vi "UDP Multicast Sender.vi"() -> ()   [LabVIEW 2010]
doc: "Designed to work with the UDP Multicast Receiver.vi. Run the UDP Multicast Receiver.vi first.\n\nUDP multicast will allow LabVIEW to send data to a multicast group or to receive data sent to a multicast group. In LabVIEW, UDP multicast is used in very much the same way as UDP. The main difference is there are two new parameters, TTL and Multicast Address, on the UDP Multicast Open. \n\nWhen sending to a multicast group the default time-to-live (TTL) is 1, which only allows the packet to go to the local subnet. When a router receives a multicast packet, it decrements the packets TTL, and if the TTL is greater than 0, forwards the packet to other routers.\nA multicast group is defined by having a multicast IP address in the range 224.0.0.0 to 239.255.255.255."
uses:
  <vilib>/Utility/tcp.llb/UDP Multicast Open.vi
panel:
  in  "milliseconds to wait":u32=50
  in  "stop":bool
  in  "Multicast Address":string="234.5.6.7"
  in  "Data String":string="UDP Multicast Sender Data"
  in  "Send to Port":u16=58432
  in  "Local Port":u16=58431
  in  "TTL":u16=2
  # "Instructions:\n1. Open the UDP Multicast Receiver.vi located in the same library.\n2. Make sure that Remote Port in this VI and Port in the UDP Multicast Receiver.vi are the same and that they have the same Multicast Address.\n3. Follow the instructions on it's front panel.\nNote: This VI is built to work with the UDP Multicast Receiver.vi."
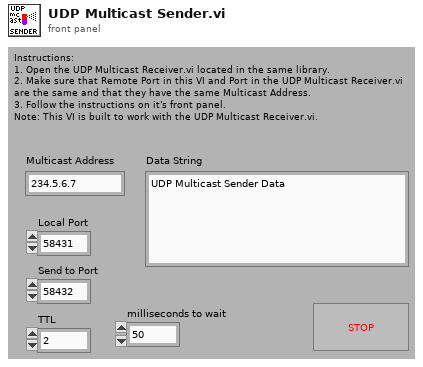
[diagram p1: front panel]
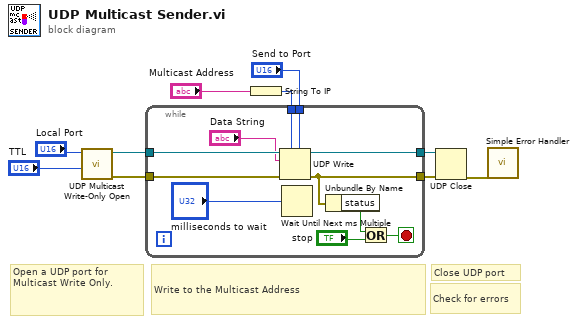
[diagram p0: block diagram]
diagram:
  # "Check for errors"
  # "Close UDP port"
  # "Write to the Multicast Address"
  # "Open a UDP port for Multicast Write Only."
  n1 = call-poly <vilib>:"UDP Multicast Write-Only Open.vi"("time-to-live (1)"="TTL", "port"="Local Port") -> ("error out"=w8:errorcluster, "connection ID"=w10:refnum<k16>)  [unwired: 8 in]
  n2 = String To IP(1:"Multicast Address") -> (0:w5:u32)
  n3 = while {
    tunnel: w10 -> [w21]
    tunnel: [w20] -> w9
    tunnel: w8 -> [w19]
    tunnel: [w12] -> w7
    tunnel: "Send to Port" -> [w18]
    tunnel: w5 -> [w17]
    stop <- w13 stop-if-true
    n4 = UDP Write(address=w17, port or service name=w18, connection ID=w21, data in="Data String", 8:w19) -> (error out=w12:errorcluster, 3:w20:refnum<k16>)  [unwired: 1 in]
    n5 = Wait Until Next ms Multiple(millisecond multiple="milliseconds to wait") -> ()  [unwired: 1 out]
    n6 = Unbundle By Name(w12) -> ("status"=w15:bool)
    n7 = Or(x=w15, y="stop") -> (x .or. y?=w13:bool)
  }
  n8 = UDP Close(connection ID=w9, 8:w7) -> (error out=w2:errorcluster)  [unwired: 1 out]
  n9 = call <vilib>:"Simple Error Handler.vi"("error in (no error)"=w2) -> ()  [unwired: 4 in, 5 out]
